vi "校准设置页.vi"() -> ()   [LabVIEW 2016, in "斯坦道CODMn.lvlib"]
uses:
  <vilib>/Analysis/6fits.llb/Curve Fitting Criteria.ctl
  <vilib>/Analysis/NI_AALPro.lvlib
  <vilib>/ptbypt/NI_PtbyPt.lvlib
panel:
  in  "读取公式":bool
  in  "历史数据导入":T1(radio)
  out "校准任务":bool
  in  "二次方程2":cluster{"K":dbl, "B":dbl, "x^2":dbl} {"x^2" format="%#.6g"; "K" format="%#.6g"; "B" format="%#.6g"}
  in  "公式切换阈值滴定数(0~9999)":dbl
  out "校准状态":T2(ring)
  out "模型刷新":bool
  in  "校准按钮":T1(radio)
  in  "校准导入":bool
  in  "曲线模型":T3={"标液浓度1"=0.0, "测量吸光度1"=0.0, "样品1启用"=FALSE, "标液浓度2"=0.0, "测量吸光度2"=0.0, "样品2启用"=FALSE, "标液浓度3"=0.0, "测量吸光度3"=0.0, "样品3启用"=FALSE, "标液浓度4"=0.0, "测量吸光度4"=0.0, "样品4启用"=FALSE, "标液浓度5"=0.0, "测量吸光度5"=0.0, "样品5启用"=FALSE, "模型"=enum."线性", "精度"=4.0, "XY图"=[], "拟合公式"="", "r^2"=0.0, "标样一校准时间"=timestamp(0 s since 1904-01-01), "标样二校准时间"=timestamp(0 s since 1904-01-01), "标样三校准时间"=timestamp(0 s since 1904-01-01), "标样四校准时间"=timestamp(0 s since 1904-01-01), "标样五校准时间"=timestamp(0 s since 1904-01-01), "二次方程"={"K"=0.0, "B"=0.0, "x^2"=0.0}, "标定时间"=timestamp(0 s since 1904-01-01), "拟合公式 2"="", "r^2 2"=0.0} {"r^2 2" format="%.7f"; "标定时间" format="%<%Y/%m/%d %H:%M:%S>T"; "二次方程"."x^2" format="%#.6g"; "二次方程"."K" format="%#.6g"; "二次方程"."B" format="%#.6g"; "标样五校准时间" format="%<%Y/%m/%d %H:%M:%S>T"; "标样四校准时间" format="%<%Y/%m/%d %H:%M:%S>T"; "标样三校准时间" format="%<%Y/%m/%d %H:%M:%S>T"; "标样二校准时间" format="%<%Y/%m/%d %H:%M:%S>T"; "标样一校准时间" format="%<%Y/%m/%d %H:%M:%S>T"; "r^2" format="%.7f"; "测量吸光度5" format="%#.6f"; "测量吸光度4" format="%#.6f"; "测量吸光度3" format="%#.6f"; "测量吸光度2" format="%#.6f"; "测量吸光度1" format="%#.6f"}
  in  "测量模式":T4(ring)
  in  "参数下拉列表":u16(ring) items=["CODMn"=21]
  in  "量程下拉列表":enum16{"低量程", "高量程"}(ring)
  # "校准时间"
  # "标液浓度"
  # "滴定数"
  # "标液一"
  # "标液二"
  # "标液三"
  # "零点"
  # "跨度"
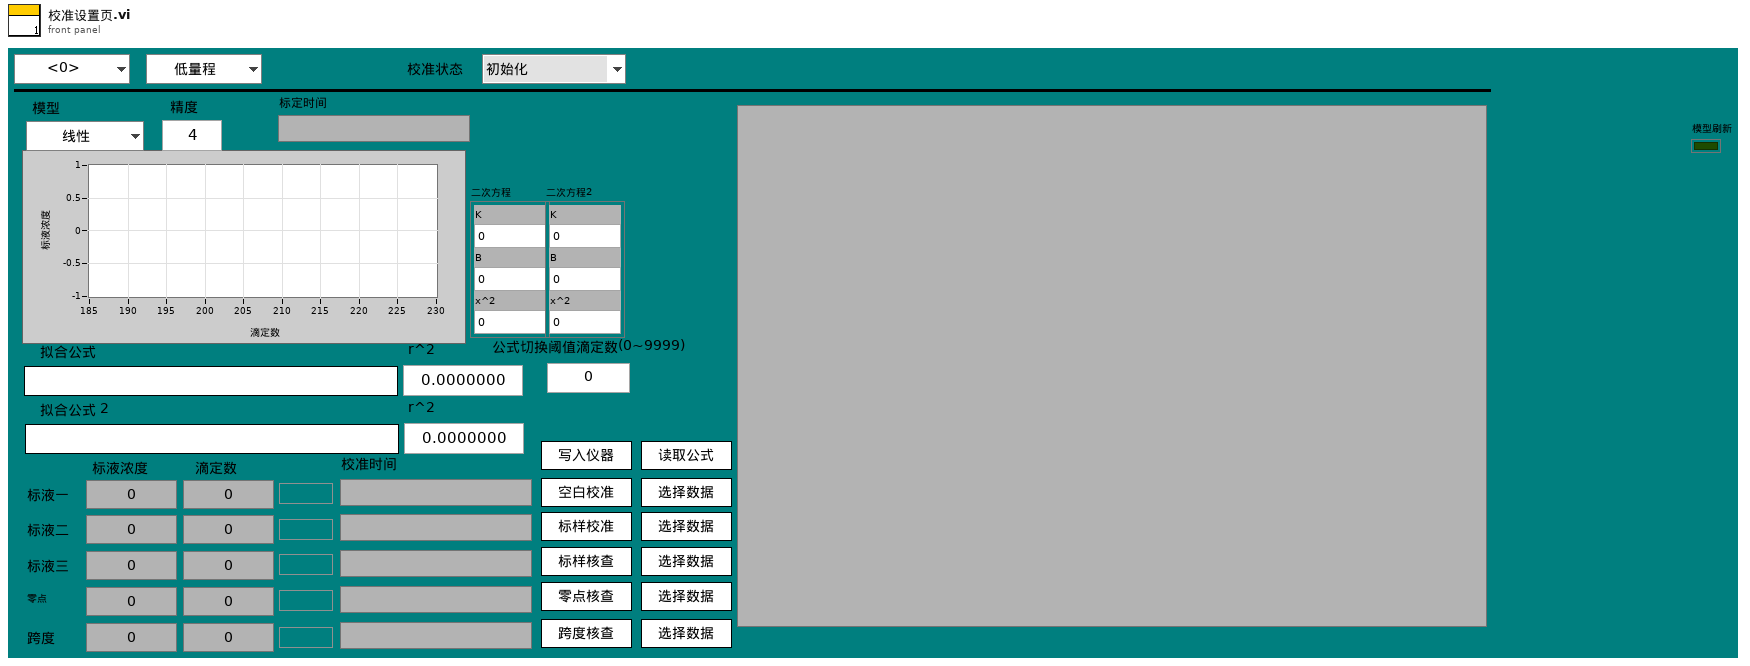
[diagram p1: front panel]
types:
  T1 = enum32{"未选择", "空白校准", "标样校准", "标样核查", "零点核查", "跨度核查"}
  T2 = enum16{"初始化", "解析数据", "判断任务类型", "执行测试任务", "等待测试任务完成", "获取测试数据", "任务结束判定", "计算公式", "结束"}
  T3 = cluster{"标液浓度1":dbl, "测量吸光度1":dbl, "样品1启用":bool, "标液浓度2":dbl, "测量吸光度2":dbl, "样品2启用":bool, "标液浓度3":dbl, "测量吸光度3":dbl, "样品3启用":bool, "标液浓度4":dbl, "测量吸光度4":dbl, "样品4启用":bool, "标液浓度5":dbl, "测量吸光度5":dbl, "样品5启用":bool, "模型":enum32{"线性", "多项式", "折线"}, "精度":dbl, "XY图":cluster{"X Values":dbl[], "Y Values":dbl[]}[], "拟合公式":string, "r^2":dbl, "标样一校准时间":timestamp, "标样二校准时间":timestamp, "标样三校准时间":timestamp, "标样四校准时间":timestamp, "标样五校准时间":timestamp, "二次方程":cluster{"K":dbl, "B":dbl, "x^2":dbl}, "标定时间":timestamp, "拟合公式 2":string, "r^2 2":dbl}
  T4 = enum16{"", "水样测量", "标样核查", "零点核查", "跨度核查", "空白测试", "平行样测试", "加标回收", "空白校准", "标样校准"}
  T5 = typedef "斯坦道CODMn.lvlib/校准任务.ctl" = cluster{"id":u16, "任务类型":enum16{"未选择", "空白校准", "标样校准", "标样核查", "零点核查", "跨度核查"}, "量程下拉列表":enum16{"低量程", "高量程"}, "状态":enum16{"已执行", "待执行", "执行中", "停止"}, "标液浓度":dbl, "吸光值":dbl, "校准时间":timestamp, "报警状态":enum16{"正常数据", "报警数据"}}
  T6 = cluster{"数组 2[0]":sgl, "数组 2[1]":sgl, "数组 2[2]":sgl, "数组 2[3]":sgl, "数组 2[4]":sgl, "数组 2[5]":sgl, "数组 2[6]":sgl, "数组 2[7]":sgl, "数组 2[8]":sgl, "数组 2[9]":sgl, "数组 2[10]":sgl, "数组 2[11]":sgl, "数组 2[12]":sgl, "数组 2[13]":sgl, "数组 2[14]":sgl, "数组 2[15]":sgl, "数组 2[16]":sgl, "数组 2[17]":sgl, "数组 2[18]":sgl, "数组 2[19]":sgl, "数组 2[20]":sgl, "数组 2[21]":sgl, "数组 2[22]":sgl, "数组 2[23]":sgl, "数组 2[24]":sgl, "数组 2[25]":sgl, "数组 2[26]":sgl, "数组 2[27]":sgl, "数组 2[28]":sgl, "数组 2[29]":sgl, "数组 2[30]":sgl, "数组 2[31]":sgl, "数组 2[32]":sgl, "数组 2[33]":sgl, "数组 2[34]":sgl, "数组 2[35]":sgl, "数组 2[36]":sgl, "数组 2[37]":sgl, "数组 2[38]":sgl, "数组 2[39]":sgl, "数组 2[40]":sgl, "数组 2[41]":sgl}
  T7 = cluster{"标液浓度1":dbl, "测量吸光度1":dbl, "样品1启用":bool, "标液浓度2":dbl, "测量吸光度2":dbl, "样品2启用":bool, "标液浓度3":dbl, "测量吸光度3":dbl, "样品3启用":bool, "标液浓度4":dbl, "测量吸光度4":dbl, "样品4启用":bool, "标液浓度5":dbl, "测量吸光度5":dbl, "样品5启用":bool, "模型":enum32{"线性", "多项式", "折线"}, "精度":dbl, "XY图":cluster{"X Values":dbl[], "Y Values":dbl[]}[], "拟合公式":string, "r^2":dbl, "标样一校准时间":timestamp, "标样二校准时间":timestamp, "标样三校准时间":timestamp, "标样四校准时间":timestamp, "标样五校准时间":timestamp, "二次方程":cluster{"c":dbl, "x":dbl, "x^2":dbl}, "标定时间":timestamp, "拟合公式 2":string, "r^2 2":dbl}[][]
  T8 = cluster{"标液浓度1":dbl, "测量吸光度1":dbl, "样品1启用":bool, "标液浓度2":dbl, "测量吸光度2":dbl, "样品2启用":bool, "标液浓度3":dbl, "测量吸光度3":dbl, "样品3启用":bool, "标液浓度4":dbl, "测量吸光度4":dbl, "样品4启用":bool, "标液浓度5":dbl, "测量吸光度5":dbl, "样品5启用":bool, "模型":enum32{"线性", "多项式", "折线"}, "精度":dbl, "XY图":cluster{"X Values":dbl[], "Y Values":dbl[]}[], "拟合公式":string, "r^2":dbl, "标样一校准时间":timestamp, "标样二校准时间":timestamp, "标样三校准时间":timestamp, "标样四校准时间":timestamp, "标样五校准时间":timestamp, "二次方程":cluster{"c":dbl, "x":dbl, "x^2":dbl}, "标定时间":timestamp, "拟合公式 2":string, "r^2 2":dbl}
  T9 = typedef "NI_AALPro.lvlib/Curve Fitting Criteria.ctl" = u16
  T10 = enum32{"Bad", "Idle", "Run top level", "Running"}
  T11 = cluster{"时间":timestamp, "标液值":dbl, "检测值":dbl, "吸光值":dbl}
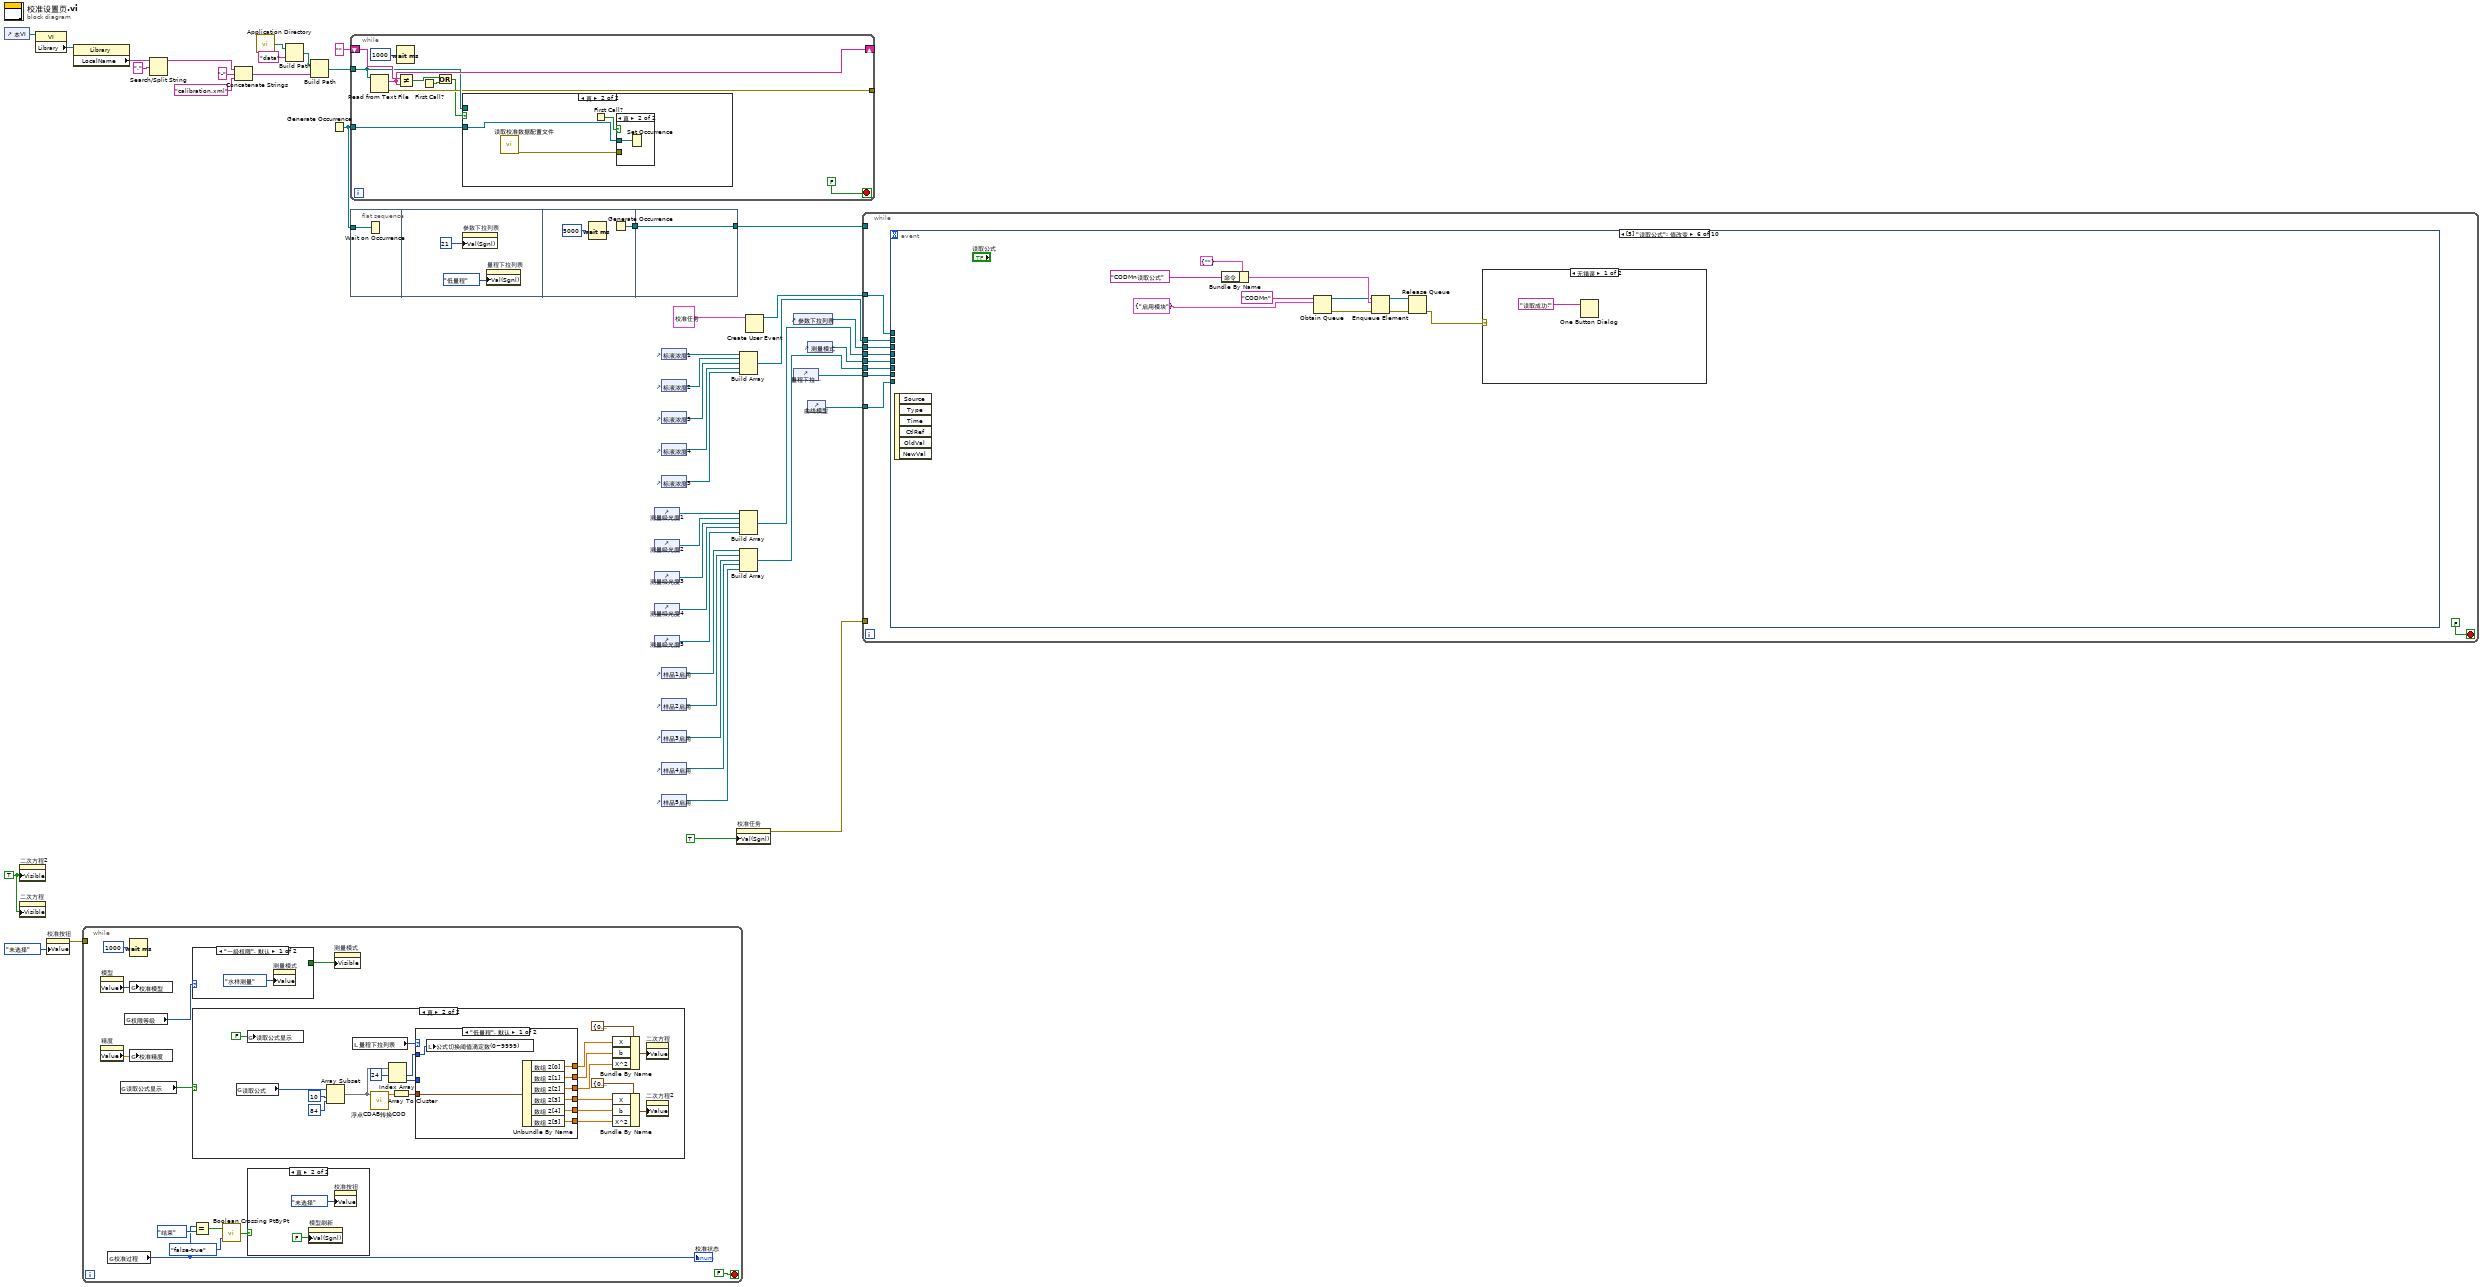
[diagram p0: block diagram]
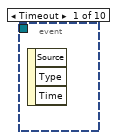
[diagram p4: hidden frame]
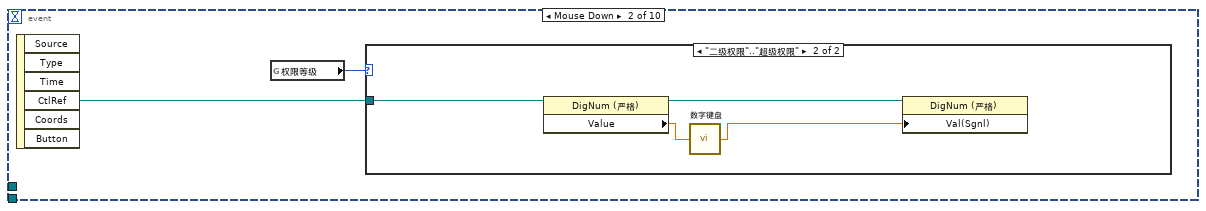
[diagram p5: hidden frame]
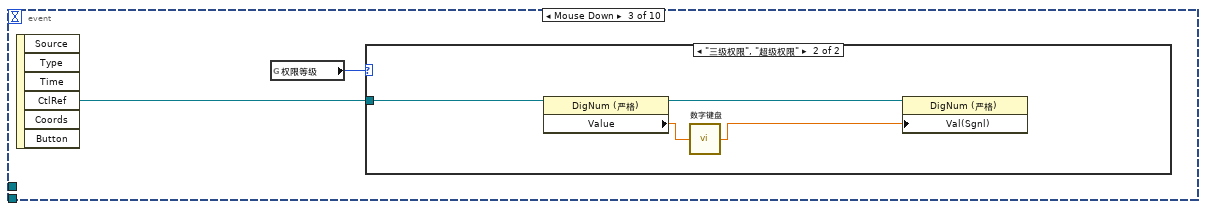
[diagram p7: hidden frame]
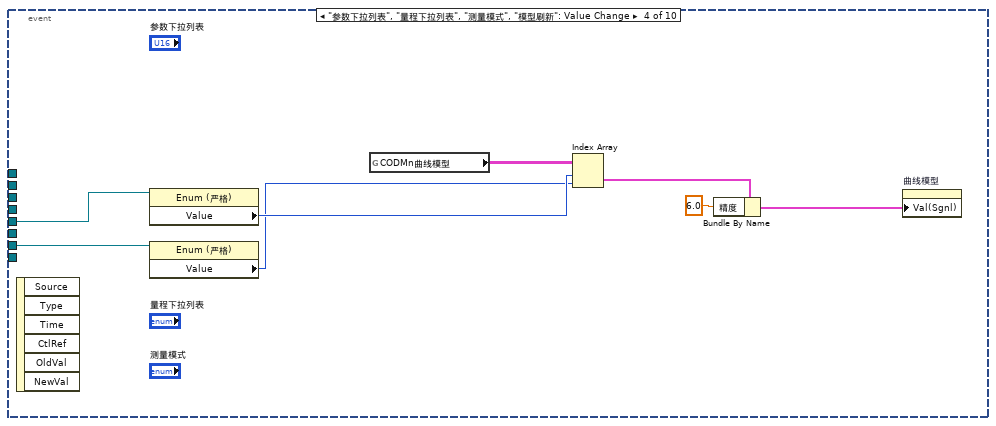
[diagram p9: hidden frame]
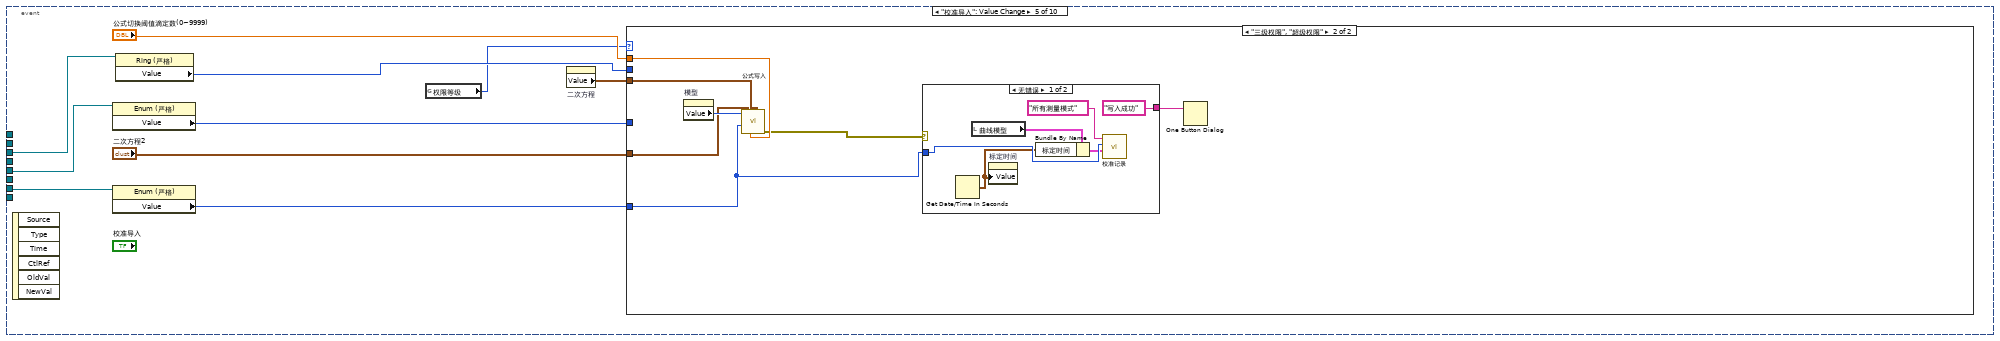
[diagram p10: hidden frame]
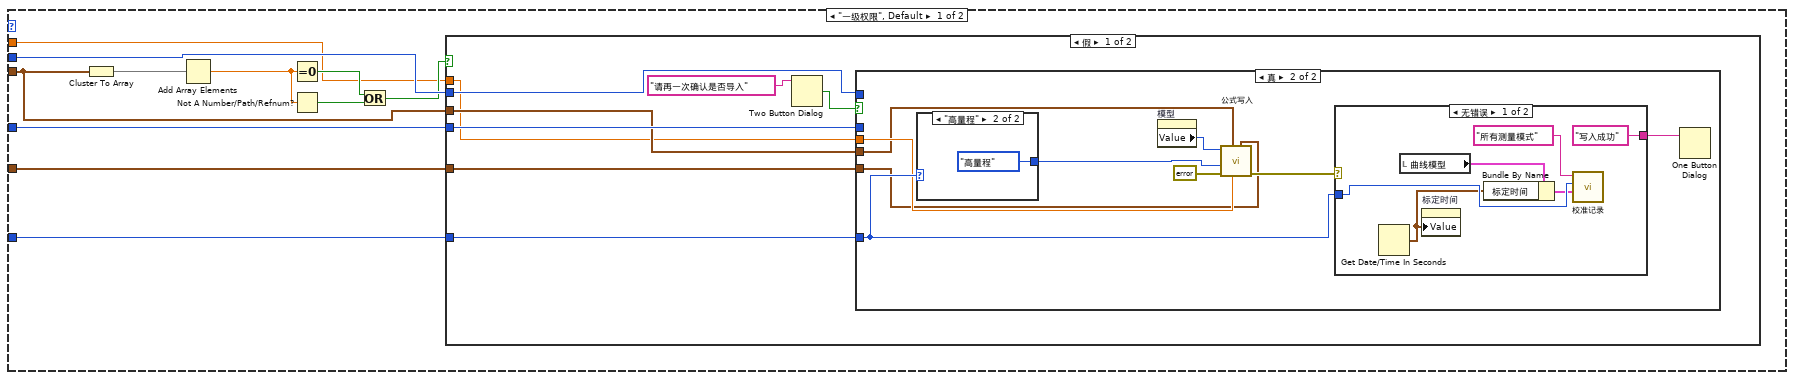
[diagram p11: hidden frame]
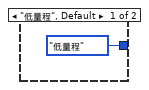
[diagram p13: hidden frame]
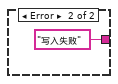
[diagram p14: hidden frame]
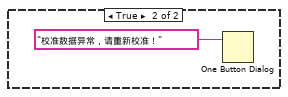
[diagram p15: hidden frame]
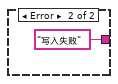
[diagram p16: hidden frame]
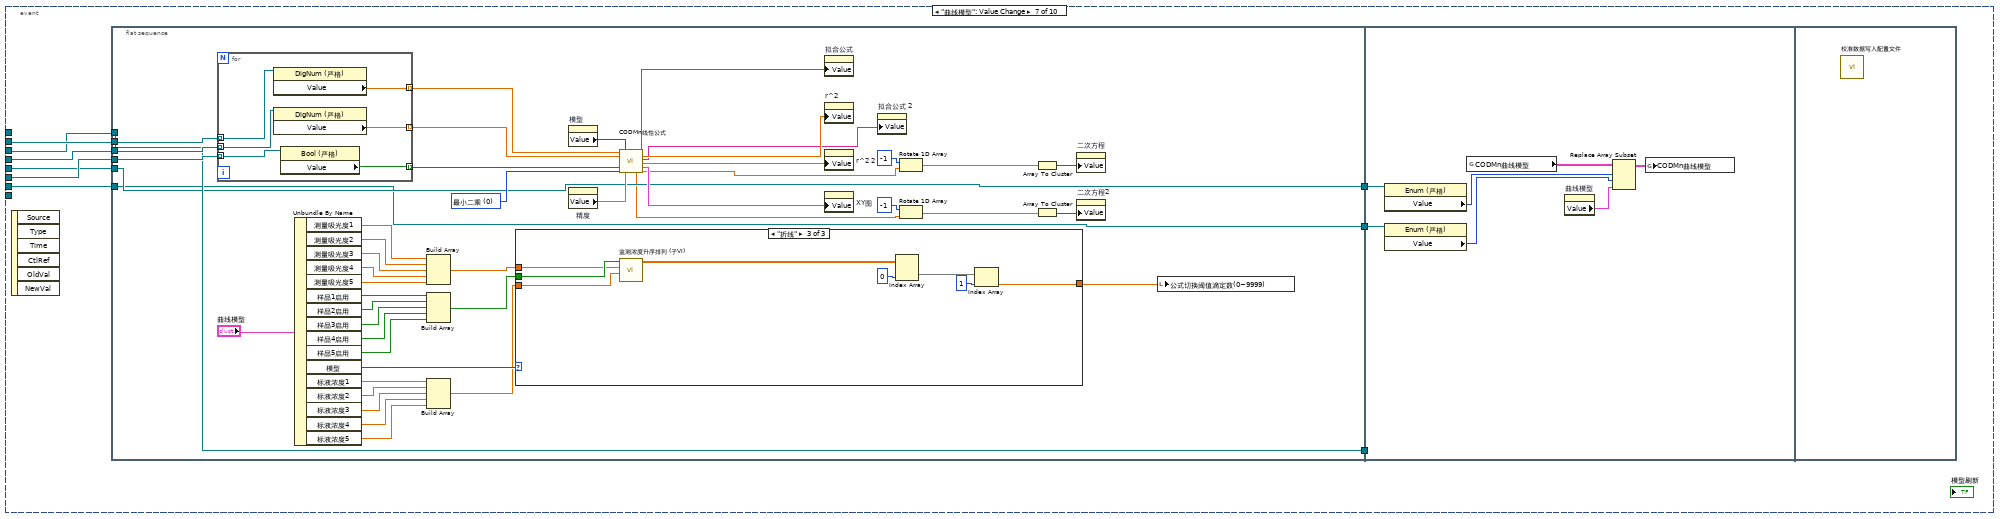
[diagram p18: hidden frame]
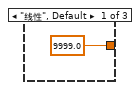
[diagram p19: hidden frame]
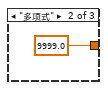
[diagram p20: hidden frame]
diagram:
  w2 = TRUE ("可见")
  n1 = control-ref of="本VI"() -> (w9:refnum<vi>)
  n2 = property on="二次方程2" class="Clust (严格)"("Visible"=w2) -> ()  [unwired: 2 in, 2 out]
  n3 = property on="二次方程" class="Clust (严格)"("Visible"=w2) -> ()  [unwired: 2 in, 2 out]
  n4 = property class="VI"(reference=w9) -> ("Library"=w18:refnum<vi>)  [unwired: 1 in, 2 out]
  n5 = property on="校准按钮" class="RadioBtnsControl (严格)"("Value"=T1."未选择" ("校准按钮")) -> (error out=w1:errorcluster)  [unwired: 2 in, 1 out]
  n6 = property class="Library"(reference=w18) -> ("LocalName"=w16:string)  [unwired: 1 in, 2 out]
  n7 = while {
    tunnel: w1 -> [_]
    stop <- FALSE stop-if-true
    n8 = property on="模型" class="Enum (严格)"() -> ("Value"=w49:enum32{"线性", "多项式", "折线"})  [unwired: 2 in, 2 out]
    n9 = property on="精度" class="DigNum (严格)"() -> ("Value"=w48:dbl)  [unwired: 2 in, 2 out]
    n10 = global read "校准数据全局变量.vi" "校准过程"() -> (w50:T2)
    "校准状态" <- w50
    n11 = global read "COD内部交互全局.vi" "读取公式显示"() -> (w46:bool)
    n12 = global read "CODMN外部API.vi" "权限等级"() -> (w47:enum16{"一级权限", "二级权限", "三级权限", "超级权限"})
    n13 = Wait (ms)(milliseconds to wait=u32 1000 ("等待时间（毫秒）")) -> ()  [unwired: 1 out]
    n14 = global write "校准数据全局变量.vi" "校准模型"(w49) -> ()
    n15 = global write "校准数据全局变量.vi" "校准精度"(w48) -> ()
    n16 = case shown="\"一级权限\", 默认" w47 {
      tunnel: [_ TRUE ("可见")] -> w55
      frame "一级权限", Default {
        n17 = property on="测量模式" class="Enum (严格)"("Value"=T4."水样测量" ("测量模式")) -> ()  [unwired: 2 in, 2 out]
      }
      frame "三级权限", "超级权限" {
      }
    }
    n18 = case shown="真" w46 {
      frame False {
      }
      frame True {
        n19 = global read "COD内部交互全局.vi" "读取公式"() -> (w72:u16[])
        n20 = global write "COD内部交互全局.vi" "读取公式显示"(FALSE ("读取公式显示")) -> ()
        n21 = Array Subset(array=w72, index=10 ("索引"), length=84 ("长度")) -> (w74:u16[])
        n22 = local read "量程下拉列表"() -> (w71:enum16{"低量程", "高量程"})
        n23 = call "浮点CDAB转换COD.vi"("数组"=w74) -> ("数组 2"=w77:sgl[])  [unwired: 10 in]
        n24 = Index Array(array=w74, index #1=24 ("索引")) -> (element #1=w68:u16, element #2=w69:u16)  [unwired: 1 in]
        n25 = Array To Cluster(array=w77) -> (cluster=w70:T6)
        n26 = case shown="\"低量程\", 默认" w71 {
          tunnel: w70 -> [w86 w93]
          tunnel: w69 -> [_ w94]
          tunnel: w68 -> [w85 _]
          tunnel: [w84 w92] -> w65
          tunnel: [w83 w91] -> w64
          tunnel: [w82 w90] -> w63
          tunnel: [w81 w89] -> w62
          tunnel: [w80 w88] -> w61
          tunnel: [w79 w87] -> w60
          frame "低量程", Default {
            n27 = local write "公式切换阈值滴定数(0~9999)"(w85) -> ()
            n28 = Unbundle By Name(w86) -> ("数组 2[0]"=w84:sgl, "数组 2[1]"=w83:sgl, "数组 2[2]"=w82:sgl, "数组 2[3]"=w81:sgl, "数组 2[4]"=w80:sgl, "数组 2[5]"=w79:sgl)
          }
          frame "高量程" {
            n29 = local write "公式切换阈值滴定数(0~9999)"(w94) -> ()
            n30 = Unbundle By Name(w93) -> ("数组 2[6]"=w92:sgl, "数组 2[7]"=w91:sgl, "数组 2[8]"=w90:sgl, "数组 2[9]"=w89:sgl, "数组 2[10]"=w88:sgl, "数组 2[11]"=w87:sgl)
          }
        }
        n31 = Bundle By Name(cluster=cluster{"X":dbl, "b":dbl, "X^2":dbl} {"X"=0.0, "b"=0.0, "X^2"=0.0} ("方程系数"), "X"=w65, "b"=w64, "X^2"=w63) -> (w59:cluster{"X":dbl, "b":dbl, "X^2":dbl})
        n32 = Bundle By Name(cluster=cluster{"X":dbl, "b":dbl, "X^2":dbl} {"X"=0.0, "b"=0.0, "X^2"=0.0} ("方程系数"), "X"=w62, "b"=w61, "X^2"=w60) -> (w58:cluster{"X":dbl, "b":dbl, "X^2":dbl})
        n33 = property on="二次方程" class="Clust (严格)"("Value"=w59) -> ()  [unwired: 2 in, 2 out]
        n34 = property on="二次方程2" class="Clust (严格)"("Value"=w58) -> ()  [unwired: 2 in, 2 out]
      }
    }
    n35 = Equal?(x=w50, y=T2."结束" ("校准过程")) -> (x = y?=w54:bool)
    n36 = call <vilib>:"Boolean Crossing PtByPt.vi"("direction"=enum16{"either", "false-true", "true-false"}."false-true", "input"=w54) -> ("crossing"=w52:bool)  [unwired: 1 in]
    n37 = case shown="真" w52 {
      frame False {
      }
      frame True {
        n38 = property on="模型刷新" class="Bool (严格)"("Val(Sgnl)"=FALSE ("值(信号)")) -> ()  [unwired: 2 in, 2 out]
        n39 = property on="校准按钮" class="RadioBtnsControl (严格)"("Value"=T1."未选择" ("校准按钮")) -> ()  [unwired: 2 in, 2 out]
      }
    }
    n40 = property on="测量模式" class="Enum (严格)"("Visible"=w55) -> ()  [unwired: 2 in, 2 out]
  }
  n41 = Search/Split String(string=w16, search string/char (-)="." ("搜索字符串/字符(-)")) -> (substring before match=w14:string)  [unwired: 1 in, 2 out]
  n42 = Concatenate Strings(w14, "-" ("字符串"), "calibration.xml" ("名称或相对路径")) -> (w11:string)
  n43 = call <vilib>:"Application Directory.vi"() -> ("Application Directory"=w19:path)
  n44 = Build Path(base path=w19, name or relative path="data" ("名称或相对路径")) -> (appended path=w17:path)
  n45 = Build Path(base path=w17, name or relative path=w11) -> (appended path=w10:path)
  n46 = Generate Occurrence() -> (w7:refnum<k4>)
  n47 = while {
    shift-right: [w106] -> _
    shift-left: "" -> [w107]
    tunnel: w10 -> [w105]
    tunnel: [w103] -> _
    tunnel: w7 -> [w99]
    stop <- FALSE stop-if-true
    n48 = Read from Text File(file (use dialog)=w105) -> (text=w106:string, error out=w103:errorcluster)  [unwired: 3 in, 2 out]
    n49 = Wait (ms)(milliseconds to wait=u32 1000 ("等待时间（毫秒）")) -> ()  [unwired: 1 out]
    n50 = Not Equal?(x=w107, y=w106) -> (x != y?=w101:bool)
    n51 = First Call?() -> (First Call?: T/F=w102:bool)
    n52 = Or(x=w101, y=w102) -> (x .or. y?=w100:bool)
    n53 = case shown="真" w100 {
      tunnel: w105 -> [_ _]
      tunnel: w99 -> [_ w110]
      frame False {
      }
      frame True {
        n54 = call "读取校准数据配置文件.vi"() -> ("错误输出"=w109:errorcluster)  [unwired: 11 in]
        n55 = First Call?() -> (First Call?: T/F=w111:bool)
        n56 = case shown="真" w111 {
          tunnel: w110 -> [_ w112]
          tunnel: w109 -> [_ _]
          frame False {
          }
          frame True {
            n57 = Set Occurrence(w112) -> ()
          }
        }
      }
    }
  }
  n58 = flat-sequence {
    tunnel: w7 -> [w113]
    tunnel: [w117] -> w45
    tunnel: [w118] -> w44
    tunnel: w45 -> [w118]
    frame #0 {
      n59 = Wait on Occurrence(2:w113) -> ()  [unwired: 2 in, 1 out]
    }
    frame #1 {
      n60 = property on="参数下拉列表" class="Ring (严格)"("Val(Sgnl)"=u16 21 ("值(信号)")) -> ()  [unwired: 2 in, 2 out]
      n61 = property on="量程下拉列表" class="Enum (严格)"("Val(Sgnl)"=enum16{"低量程", "高量程"}."低量程" ("值(信号)")) -> ()  [unwired: 2 in, 2 out]
    }
    frame #2 {
      n62 = Wait (ms)(milliseconds to wait=u32 5000 ("等待时间（毫秒）")) -> ()  [unwired: 1 out]
      n63 = Generate Occurrence() -> (w117:refnum<k4>)
    }
    frame #3 {
    }
  }
  n64 = control-ref of="测量吸光度1"() -> (w32:refnum<vi>)
  n65 = control-ref of="测量吸光度2"() -> (w33:refnum<vi>)
  n66 = control-ref of="测量吸光度3"() -> (w34:refnum<vi>)
  n67 = control-ref of="测量吸光度4"() -> (w35:refnum<vi>)
  n68 = control-ref of="测量吸光度5"() -> (w36:refnum<vi>)
  n69 = control-ref of="标液浓度1"() -> (w30:refnum<vi>)
  n70 = control-ref of="标液浓度2"() -> (w29:refnum<vi>)
  n71 = control-ref of="标液浓度3"() -> (w28:refnum<vi>)
  n72 = control-ref of="标液浓度4"() -> (w27:refnum<vi>)
  n73 = control-ref of="标液浓度5"() -> (w26:refnum<vi>)
  n74 = control-ref of="样品1启用"() -> (w42:refnum<vi>)
  n75 = control-ref of="样品2启用"() -> (w41:refnum<vi>)
  n76 = control-ref of="样品3启用"() -> (w40:refnum<vi>)
  n77 = control-ref of="样品4启用"() -> (w39:refnum<vi>)
  n78 = control-ref of="样品5启用"() -> (w38:refnum<vi>)
  n79 = property on="校准任务" class="Bool (严格)"("Val(Sgnl)"=TRUE ("值(信号)")) -> (error out=w5:errorcluster)  [unwired: 2 in, 1 out]
  n80 = Build Array(w30, w29, w28, w27, w26) -> (w25:refnum<vi>[])
  n81 = Build Array(w32, w33, w34, w35, w36) -> (w31:refnum<vi>[])
  n82 = Build Array(w42, w41, w40, w39, w38) -> (w37:refnum<vi>[])
  n83 = Create User Event(user event datatype=T5 {"id"=0, "任务类型"=enum."未选择", "量程下拉列表"=enum."低量程", "状态"=enum."已执行", "标液浓度"=0.0, "吸光值"=0.0, "校准时间"=timestamp(0 s since 1904-01-01), "报警状态"=enum."正常数据"} ("校准任务")) -> (user event=w3:refnum<user-event>)  [unwired: 1 in, 1 out]
  n84 = control-ref of="参数下拉列表"() -> (w43:refnum<vi>)
  n85 = control-ref of="量程下拉列表"() -> (w23:refnum<vi>)
  n86 = control-ref of="测量模式"() -> (w24:refnum<vi>)
  n87 = control-ref of="曲线模型"() -> (w21:refnum<vi>)
  n88 = while {
    tunnel: w44 -> [_]
    tunnel: w43 -> [w126]
    tunnel: w37 -> [w125]
    tunnel: w31 -> [w124]
    tunnel: w25 -> [w123]
    tunnel: w24 -> [w122]
    tunnel: w23 -> [w121]
    tunnel: w21 -> [w120]
    tunnel: w5 -> [_]
    tunnel: w3 -> [w119]
    stop <- FALSE stop-if-true
    n89 = event shown="[5] \"读取公式\": 值改变" {
      selector: _ -> [_ _ _ _ _ _ _ _ _ _]
      dyn-events: _ -> [_ _ _ _ _ _ _ _ _ _]
      timeout: _ -> [_ _ _ _ _ _ _ _ _ _]
      tunnel: w126 -> [_ _ _ _ w157 _ w225 _ w327 w354]
      tunnel: w125 -> [_ _ _ _ _ _ w229 _ _ _]
      tunnel: w124 -> [_ _ _ _ _ _ w228 _ _ _]
      tunnel: w123 -> [_ _ _ _ _ _ w227 _ _ _]
      tunnel: w122 -> [_ _ _ w147 w155 _ w223 _ w322 w349]
      tunnel: w121 -> [_ _ _ w146 w153 _ w221 _ w326 w353]
      tunnel: w120 -> [_ _ _ _ _ _ _ _ w320 _]
      tunnel: w119 -> [_ _ _ _ _ _ _ w300 w319 w348]
      event Timeout {
        n90 = event-data() -> ()  [unwired: 1 in, 3 out]
      }
      event "曲线模型.标液浓度1", "曲线模型.标液浓度2", "曲线模型.标液浓度3", "曲线模型.标液浓度4", "曲线模型.标液浓度5", "曲线模型.精度": Mouse Down {
        n91 = event-data() -> ("CtlRef"=w129:refnum<vi>)  [unwired: 1 in, 5 out]
        n92 = global read "CODMN外部API.vi" "权限等级"() -> (w128:enum16{"一级权限", "二级权限", "三级权限", "超级权限"})
        n93 = case shown="\"二级权限\"..\"超级权限\"" w128 {
          tunnel: w129 -> [_ w133]
          frame "一级权限", Default {
          }
          frame "二级权限".."超级权限" {
            n94 = property class="DigNum (严格)"(reference=w133) -> (reference out=w131:refnum<vi>, "Value"=w132:dbl)  [unwired: 1 in, 1 out]
            n95 = call "数字键盘.vi"("OldNumber"=w132) -> ("NewNumber"=w130:sgl)
            n96 = property class="DigNum (严格)"(reference=w131, "Val(Sgnl)"=w130) -> ()  [unwired: 1 in, 2 out]
          }
        }
      }
      event "曲线模型.测量吸光度1", "曲线模型.测量吸光度2", "曲线模型.测量吸光度3", "曲线模型.测量吸光度4", "曲线模型.测量吸光度5": Mouse Down {
        n97 = event-data() -> ("CtlRef"=w135:refnum<vi>)  [unwired: 1 in, 5 out]
        n98 = global read "CODMN外部API.vi" "权限等级"() -> (w134:enum16{"一级权限", "二级权限", "三级权限", "超级权限"})
        n99 = case shown="\"三级权限\", \"超级权限\"" w134 {
          tunnel: w135 -> [_ w139]
          frame "一级权限", Default {
          }
          frame "三级权限", "超级权限" {
            n100 = property class="DigNum (严格)"(reference=w139) -> (reference out=w137:refnum<vi>, "Value"=w138:dbl)  [unwired: 1 in, 1 out]
            n101 = call "数字键盘.vi"("OldNumber"=w138) -> ("NewNumber"=w136:sgl)
            n102 = property class="DigNum (严格)"(reference=w137, "Val(Sgnl)"=w136) -> ()  [unwired: 1 in, 2 out]
          }
        }
      }
      event "参数下拉列表", "量程下拉列表", "测量模式", "模型刷新": Value Change {
        n103 = event-data() -> ()  [unwired: 1 in, 6 out]
        n104 = property class="Enum (严格)"(reference=w147) -> ("Value"=w144:T4)  [unwired: 1 in, 2 out]
        n105 = property class="Enum (严格)"(reference=w146) -> ("Value"=w143:enum16{"低量程", "高量程"})  [unwired: 1 in, 2 out]
        n106 = global read "校准数据全局变量.vi" "CODMn曲线模型"() -> (w145:T7)
        n107 = Index Array(array=w145, index (row)=w144, index (col)=w143) -> (element=w142:T8)
        n108 = Bundle By Name(cluster=w142, "精度"=6.0 ("值")) -> (w141:T8)
        n109 = property on="曲线模型" class="Clust (严格)"("Val(Sgnl)"=w141) -> ()  [unwired: 2 in, 2 out]
      }
      event "校准导入": Value Change {
        n110 = event-data() -> ()  [unwired: 1 in, 6 out]
        n111 = property class="Enum (严格)"(reference=w155) -> ("Value"=w154:T4)  [unwired: 1 in, 2 out]
        n112 = property class="Enum (严格)"(reference=w153) -> ("Value"=w152:enum16{"低量程", "高量程"})  [unwired: 1 in, 2 out]
        n113 = property class="Ring (严格)"(reference=w157) -> ("Value"=w156:u16)  [unwired: 1 in, 2 out]
        n114 = global read "CODMN外部API.vi" "权限等级"() -> (w149:enum16{"一级权限", "二级权限", "三级权限", "超级权限"})
        n115 = property on="二次方程" class="Clust (严格)"() -> ("Value"=w148:cluster{"K":dbl, "B":dbl, "x^2":dbl})  [unwired: 2 in, 2 out]
        n116 = case shown="\"三级权限\", \"超级权限\"" w149 {
          tunnel: w156 -> [w168 _]
          tunnel: w154 -> [w167 _]
          tunnel: w152 -> [w166 w196]
          tunnel: w148 -> [w160 w200]
          tunnel: "公式切换阈值滴定数(0~9999)" -> [w159 w201]
          tunnel: "二次方程2" -> [w158 w199]
          frame "一级权限", Default {
            n117 = Cluster To Array(cluster=w160) -> (array=w165:dbl[])
            n118 = Add Array Elements(numeric array=w165) -> (sum=w164:dbl)
            n119 = Equal To 0?(x=w164) -> (x = 0?=w162:bool)
            n120 = Not A Number/Path/Refnum?(number/path/refnum=w164) -> (NaN/Path/Refnum?=w163:bool)
            n121 = Or(x=w162, y=w163) -> (x .or. y?=w161:bool)
            n122 = case shown="假" w161 {
              tunnel: w168 -> [w176 _]
              tunnel: w167 -> [w175 _]
              tunnel: w166 -> [w174 _]
              tunnel: w160 -> [w171 _]
              tunnel: w159 -> [w170 _]
              tunnel: w158 -> [w169 _]
              frame False {
                n123 = Two Button Dialog(message="请再一次确认是否导入" ("消息")) -> (T button?=w172:bool)  [unwired: 2 in]
                n124 = case shown="真" w172 {
                  tunnel: w176 -> [_ _]
                  tunnel: w175 -> [_ _]
                  tunnel: w174 -> [_ w184]
                  tunnel: w171 -> [_ w177]
                  tunnel: w170 -> [_ w180]
                  tunnel: w169 -> [_ w178]
                  frame False {
                  }
                  frame True {
                    n125 = case shown="\"高量程\"" w184 {
                      tunnel: [enum16{"低量程", "高量程"}."低量程" ("量程选择") enum16{"低量程", "高量程"}."高量程" ("量程选择")] -> w181
                      frame "低量程", Default {
                      }
                      frame "高量程" {
                      }
                    }
                    n126 = property on="模型" class="Enum (严格)"() -> ("Value"=w179:enum32{"线性", "多项式", "折线"})  [unwired: 2 in, 2 out]
                    n127 = call "公式写入.vi"("公式 2"=w178, "公式切换阈值滴定数(0-9999)"=w180, "公式"=w177, "Error in"=errorcluster {"status"=FALSE, "code"=0, "source"=""} ("error out"), "量程选择"=w181, "模型"=w179) -> ("error out"=w183:errorcluster)  [unwired: 5 in]
                    n128 = case shown="无错误" w183 {
                      tunnel: ["写入成功" "写入失败"] -> w185
                      tunnel: w184 -> [w192 _]
                      frame No Error {
                        n129 = Get Date/Time In Seconds() -> (seconds since 1Jan1904=w189:timestamp)
                        n130 = local read "曲线模型"() -> (w190:T3)
                        n131 = property on="标定时间" class="AbsTime (严格)"("Value"=w189) -> ()  [unwired: 2 in, 2 out]
                        n132 = Bundle By Name(cluster=w190, "标定时间"=w189) -> (w188:T3)
                        n133 = call "校准记录.vi"("曲线模型"=w188, "量程"=w192, "测量模式"="所有测量模式") -> ()  [unwired: 8 in, 1 out]
                      }
                      frame Error {
                      }
                    }
                    n134 = One Button Dialog(message=w185) -> ()  [unwired: 1 in, 1 out]
                  }
                }
              }
              frame True {
                n135 = One Button Dialog(message="校准数据异常，请重新校准！" ("消息")) -> ()  [unwired: 1 in, 1 out]
              }
            }
          }
          frame "三级权限", "超级权限" {
            n136 = property on="模型" class="Enum (严格)"() -> ("Value"=w202:enum32{"线性", "多项式", "折线"})  [unwired: 2 in, 2 out]
            n137 = call "公式写入.vi"("公式 2"=w199, "公式切换阈值滴定数(0-9999)"=w201, "公式"=w200, "量程选择"=w196, "模型"=w202) -> ("error out"=w197:errorcluster)  [unwired: 6 in]
            n138 = case shown="无错误" w197 {
              tunnel: ["写入成功" "写入失败"] -> w198
              tunnel: w196 -> [w207 _]
              frame No Error {
                n139 = Get Date/Time In Seconds() -> (seconds since 1Jan1904=w204:timestamp)
                n140 = local read "曲线模型"() -> (w205:T3)
                n141 = property on="标定时间" class="AbsTime (严格)"("Value"=w204) -> ()  [unwired: 2 in, 2 out]
                n142 = Bundle By Name(cluster=w205, "标定时间"=w204) -> (w203:T3)
                n143 = call "校准记录.vi"("曲线模型"=w203, "量程"=w207, "测量模式"="所有测量模式") -> ()  [unwired: 8 in, 1 out]
              }
              frame Error {
              }
            }
            n144 = One Button Dialog(message=w198) -> ()  [unwired: 1 in, 1 out]
          }
        }
      }
      event "读取公式": Value Change {
        n145 = event-data() -> ()  [unwired: 1 in, 6 out]
        n146 = Bundle By Name(cluster=cluster{"命令":string} {"命令"=""} ("元素"), "命令"="CODMn读取公式" ("名称（未命名）")) -> (w217:cluster{"命令":string})
        n147 = Obtain Queue(name (unnamed)="CODMn" ("名称（未命名）"), element data type=cluster{"命令":string} {"命令"="启用模块"} ("元素")) -> (queue out=w213:refnum<queue>, error out=w214:errorcluster)  [unwired: 3 in, 1 out]
        n148 = Enqueue Element(queue=w213, element=w217, error in (no error)=w214) -> (queue out=w212:refnum<queue>, error out=w211:errorcluster)  [unwired: 1 in, 1 out]
        n149 = Release Queue(queue=w212, error in (no error)=w211) -> (error out=w210:errorcluster)  [unwired: 1 in, 2 out]
        n150 = case shown="无错误" w210 {
          frame No Error {
            n151 = One Button Dialog(message="读取成功!") -> ()  [unwired: 1 in, 1 out]
          }
          frame Error {
          }
        }
      }
      event "曲线模型": Value Change {
        n152 = event-data() -> ()  [unwired: 1 in, 6 out]
        n153 = flat-sequence {
          tunnel: w229 -> [w275]
          tunnel: w228 -> [w273]
          tunnel: w227 -> [w271]
          tunnel: [w263] -> w226
          tunnel: w225 -> [w263]
          tunnel: [w262] -> w224
          tunnel: w223 -> [w262]
          tunnel: [w261] -> w222
          tunnel: w221 -> [w261]
          tunnel: w226 -> [_]
          tunnel: w224 -> [w297]
          tunnel: w222 -> [w296]
          frame #0 {
            w267 = T9 0 items=["最小二乘", "最小绝对残差", "Bisquare"] ("method")
            n154 = for {
              tunnel: w275 -> [w291] mode=indexing
              tunnel: [w290] -> w274 mode=indexing
              tunnel: w273 -> [w289] mode=indexing
              tunnel: [w288] -> w272 mode=indexing
              tunnel: w271 -> [w287] mode=indexing
              tunnel: [w286] -> w270 mode=indexing
              n155 = property class="DigNum (严格)"(reference=w287) -> ("Value"=w286:dbl)  [unwired: 1 in, 2 out]
              n156 = property class="DigNum (严格)"(reference=w289) -> ("Value"=w288:dbl)  [unwired: 1 in, 2 out]
              n157 = property class="Bool (严格)"(reference=w291) -> ("Value"=w290:bool)  [unwired: 1 in, 2 out]
            }
            n158 = Unbundle By Name("曲线模型") -> ("测量吸光度1"=w259:dbl, "测量吸光度2"=w258:dbl, "测量吸光度3"=w257:dbl, "测量吸光度4"=w255:dbl, "测量吸光度5"=w256:dbl, "样品1启用"=w254:bool, "样品2启用"=w253:bool, "样品3启用"=w252:bool, "样品4启用"=w251:bool, "样品5启用"=w250:bool, "模型"=w244:enum32{"线性", "多项式", "折线"}, "标液浓度1"=w243:dbl, "标液浓度2"=w242:dbl, "标液浓度3"=w241:dbl, "标液浓度4"=w240:dbl, "标液浓度5"=w239:dbl)
            n159 = Build Array(w259, w258, w257, w255, w256) -> (w248:dbl[])
            n160 = Build Array(w254, w253, w252, w251, w250) -> (w249:bool[])
            n161 = Build Array(w243, w242, w241, w240, w239) -> (w238:dbl[])
            n162 = case shown="\"折线\"" w244 {
              tunnel: w249 -> [_ _ w283]
              tunnel: w248 -> [_ _ w282]
              tunnel: [9999.0 ("数值") 9999.0 ("数值") w284] -> w245
              tunnel: w238 -> [_ _ w281]
              frame "线性", Default {
              }
              frame "多项式" {
              }
              frame "折线" {
                n163 = call "监测浓度升序排列 (子VI).vi"("标液浓度"=w281, "滴定数"=w282, "启用"=w283) -> ("输出数组"=w280:dbl[][])  [unwired: 8 in]
                n164 = Index Array(array=w280, index (col)=0 ("禁用的索引 (列)")) -> (element=w278:dbl[])  [unwired: 1 in]
                n165 = Index Array(array=w278, index=1 ("索引")) -> (element=w284:dbl)
              }
            }
            n166 = property on="模型" class="Enum (严格)"() -> ("Value"=w269:enum32{"线性", "多项式", "折线"})  [unwired: 2 in, 2 out]
            n167 = property on="精度" class="DigNum (严格)"() -> ("Value"=w268:dbl)  [unwired: 2 in, 2 out]
            n168 = call "CODMn线性公式.vi"("标液浓度"=w270, "滴定数"=w272, "启用"=w274, "method"=w267, "模型"=w269, "精度"=w268) -> ("Polynomial Coefficients 2"=w235:dbl[], "拟合方程"=w266:string, "r^2"=w265:dbl, "拟合方程 2"=w247:string, "r^2 2"=w246:dbl, "XY图"=w264:cluster{"X Values":dbl[], "Y Values":dbl[]}[], "Polynomial Coefficients"=w231:dbl[])  [unwired: 7 in]
            n169 = property on="拟合公式" class="Str"("Value"=w266) -> ()  [unwired: 2 in, 2 out]
            n170 = property on="r^2" class="DigNum (严格)"("Value"=w265) -> ()  [unwired: 2 in, 2 out]
            n171 = property on="r^2 2" class="DigNum (严格)"("Value"=w246) -> ()  [unwired: 2 in, 2 out]
            n172 = property on="XY图" class="XYGraph (严格)"("Value"=w264) -> ()  [unwired: 2 in, 2 out]
            n173 = property on="拟合公式 2" class="Str"("Value"=w247) -> ()  [unwired: 2 in, 2 out]
            n174 = Rotate 1D Array(1:w231, 2:-1 ("n")) -> (0:w233:dbl[])
            n175 = Rotate 1D Array(1:w235, 2:-1 ("n")) -> (0:w237:dbl[])
            n176 = Array To Cluster(array=w233) -> (cluster=w230:cluster{"[0]":dbl, "[1]":dbl, "[2]":dbl})
            n177 = Array To Cluster(array=w237) -> (cluster=w234:cluster{"[0]":dbl, "[1]":dbl, "[2]":dbl})
            n178 = property on="二次方程" class="Clust (严格)"("Value"=w230) -> ()  [unwired: 2 in, 2 out]
            n179 = property on="二次方程2" class="Clust (严格)"("Value"=w234) -> ()  [unwired: 2 in, 2 out]
            n180 = local write "公式切换阈值滴定数(0~9999)"(w245) -> ()
          }
          frame #1 {
            n181 = property class="Enum (严格)"(reference=w297) -> ("Value"=w294:T4)  [unwired: 1 in, 2 out]
            n182 = property class="Enum (严格)"(reference=w296) -> ("Value"=w295:enum16{"低量程", "高量程"})  [unwired: 1 in, 2 out]
            n183 = global read "校准数据全局变量.vi" "CODMn曲线模型"() -> (w293:T7)
            n184 = property on="曲线模型" class="Clust (严格)"() -> ("Value"=w298:T3)  [unwired: 2 in, 2 out]
            n185 = Replace Array Subset(array=w293, new element=w298, index (row)=w294, index (col)=w295) -> (w292:T7)
            n186 = global write "校准数据全局变量.vi" "CODMn曲线模型"(w292) -> ()
          }
          frame #2 {
            n187 = call "校准数据写入配置文件.vi"() -> ()  [unwired: 11 in, 1 out]
          }
        }
      }
      event "校准任务": Value Change {
        n188 = event-data() -> ("NewVal"=w301:bool)  [unwired: 1 in, 5 out]
        n189 = invoke on="子面板" class="SubPnl" method="Remove VI"() -> (error out=w299:errorcluster)  [unwired: 3 in, 2 out]
        n190 = case shown="真" w301 {
          tunnel: w300 -> [_ w305]
          tunnel: w299 -> [_ w302]
          frame False {
          }
          frame True {
            n191 = vi-ref "校准任务设置.vi"() -> (w308:refnum<vi>)
            n192 = property class="VI"(reference=w308) -> (reference out=w304:refnum<vi>, "Name"=w306:string, "Exec.State"=w307:T10)  [unwired: 1 in, 1 out]
            n193 = case shown="\"Idle\"" w307 {
              tunnel: w306 -> [_ w318]
              tunnel: w305 -> [_ w313]
              tunnel: w304 -> [w309 w310]
              tunnel: [w309 w310] -> w303
              frame "Bad", Default {
              }
              frame "Idle" {
                n194 = Open VI Reference(type specifier VI Refnum (for type only)=refnum<vi> refnum ("类型说明符VI引用句柄（仅用于类型）"), vi path=w318, options=128 ("选项")) -> (vi reference=w315:refnum<vi>, error out=w314:errorcluster)  [unwired: 3 in]
                n195 = call-by-ref "开始异步调用"(reference=w315, error in=w314, "用户事件"=w313) -> (reference out=w312:refnum<vi>, error out=w311:errorcluster)  [unwired: 11 in]
                n196 = Close Reference(reference=w312, error in (no error)=w311) -> ()  [unwired: 1 out]
              }
            }
            n197 = invoke on="子面板" class="SubPnl" method="Insert VI"(error in=w302, "VI Ref"=w303) -> ()  [unwired: 2 in, 4 out]
          }
        }
      }
      event "校准按钮": Value Change {
        n198 = event-data() -> ("CtlRef"=w321:refnum<vi>, "NewVal"=w323:T1)  [unwired: 1 in, 4 out]
        n199 = Not Equal?(x=w323, y=T1."未选择") -> (x != y?=w324:bool)
        n200 = case shown="真" w324 {
          tunnel: w327 -> [_ w335]
          tunnel: w326 -> [_ w333]
          tunnel: w323 -> [_ w337]
          tunnel: w322 -> [_ _]
          tunnel: w321 -> [_ _]
          tunnel: w320 -> [_ _]
          tunnel: w319 -> [_ w336]
          frame False {
          }
          frame True {
            (unwired) u16 21 items=["CODMn"=21] ("参数下拉列表")
            n201 = property class="Enum (严格)"(reference=w333) -> ("Value"=w332:enum16{"低量程", "高量程"})  [unwired: 1 in, 2 out]
            n202 = property class="Ring (严格)"(reference=w335) -> ("Value"=w334:u16)  [unwired: 1 in, 2 out]
            n203 = local read "曲线模型"() -> (w330:T3)
            n204 = case shown="\"跨度核查\"" w337 {
              tunnel: w330 -> [_ w339 w341 w342 w344 w346]
              tunnel: [_ w338 w340 w343 w345 w347] -> w329
              frame "未选择", Default {
              }
              frame "空白校准" {
                n205 = Unbundle By Name(w339) -> ("标液浓度1"=w338:dbl)
              }
              frame "标样校准" {
                n206 = Unbundle By Name(w341) -> ("标液浓度2"=w340:dbl)
              }
              frame "标样核查" {
                n207 = Unbundle By Name(w342) -> ("标液浓度3"=w343:dbl)
              }
              frame "零点核查" {
                n208 = Unbundle By Name(w344) -> ("标液浓度4"=w345:dbl)
              }
              frame "跨度核查" {
                n209 = Unbundle By Name(w346) -> ("标液浓度5"=w347:dbl)
              }
            }
            n210 = Bundle By Name(cluster=T5 {"id"=0, "任务类型"=enum."未选择", "量程下拉列表"=enum."低量程", "状态"=enum."待执行", "标液浓度"=0.0, "吸光值"=0.0, "校准时间"=timestamp(0 s since 1904-01-01), "报警状态"=enum."正常数据"} ("校准任务"), "id"=w334, "任务类型"=w337, "量程下拉列表"=w332, "标液浓度"=w329) -> (w331:T5)
            n211 = Generate User Event(user event=w336, event data cluster=w331) -> ()  [unwired: 2 in, 2 out]
          }
        }
      }
      event "历史数据导入": Value Change {
        n212 = event-data() -> ("NewVal"=w350:T1)  [unwired: 1 in, 5 out]
        n213 = Not Equal?(x=w350, y=T1."未选择") -> (x != y?=w351:bool)
        n214 = case shown="真" w351 {
          tunnel: w354 -> [_ w364]
          tunnel: w353 -> [_ w363]
          tunnel: w350 -> [_ w357]
          tunnel: w349 -> [_ _]
          tunnel: w348 -> [_ w361]
          frame False {
          }
          frame True {
            n215 = property class="Enum (严格)"(reference=w363) -> ("Value"=w359:enum16{"低量程", "高量程"})  [unwired: 1 in, 2 out]
            n216 = property class="Ring (严格)"(reference=w364) -> ("Value"=w360:u16)  [unwired: 1 in, 2 out]
            n217 = property on="历史数据导入" class="RadioBtnsControl (严格)"("Value"=T1."未选择" ("历史数据导入")) -> ()  [unwired: 2 in, 2 out]
            n218 = call "校准数据选择表.vi"("历史数据导入"=w357, "量程下拉列表"=w359, "table"="CODMn") -> ("布尔"=w362:bool, "输出"=w355:T11)  [unwired: 7 in]
            n219 = case shown="真" w362 {
              tunnel: w355 -> [_ w370]
              tunnel: w361 -> [_ w374]
              tunnel: w360 -> [_ w371]
              tunnel: w359 -> [_ w369]
              tunnel: w357 -> [_ w368]
              frame False {
              }
              frame True {
                n220 = Unbundle By Name(w370) -> ("标液值"=w367:dbl, "吸光值"=w366:dbl, "时间"=w365:timestamp)
                n221 = Bundle By Name(cluster=T5 {"id"=0, "任务类型"=enum."未选择", "量程下拉列表"=enum."低量程", "状态"=enum."已执行", "标液浓度"=0.0, "吸光值"=0.0, "校准时间"=timestamp(0 s since 1904-01-01), "报警状态"=enum."正常数据"} ("事件数据"), "id"=w371, "任务类型"=w368, "量程下拉列表"=w369, "标液浓度"=w367, "吸光值"=w366, "校准时间"=w365) -> (w372:T5)
                n222 = Generate User Event(user event=w374, event data cluster=w372) -> ()  [unwired: 2 in, 2 out]
              }
            }
          }
        }
      }
    }
  }
